vi "ALTS-2015-Read Serial Number.vi"(8 "error in (no error)":errorcluster) -> (0 "error out":errorcluster, 2 "Valid Serial Number?":bool, 3 "Serial No":string)   [LabVIEW 2013]
uses:
  Controls/ALTS-2015 LV2GBL Options.ctl
  Controls/ALTS-2015 Scanner Driver Options.ctl
  Misc/Controls/File Driver States.ctl
  OPC Engine/Controls/ALTS-2015 OPC Read Registers.ctl
  OPC Engine/Controls/ALTS-2015 OPC Read Global Options.ctl
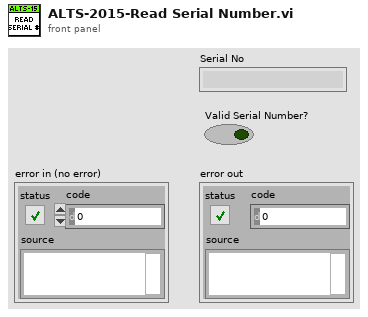
[diagram p1: front panel]
types:
  T1 = typedef "ALTS-2015 LV2GBL Options.ctl" = enum16{"Read all", "Write all"}
  T2 = typedef "ALTS-2015 INI Configuration Cluster.ctl" = cluster{"Application":cluster{"Rerun Count":i32, "Workorder No":string, "PLC Scanner":bool}, "Station Details":cluster{"Sensor Name 1":string, "Sensor Name 2":string, "Sensor Name 3":string, "Sensor Name 4":string, "Station1 Enable":bool, "Station2 Enable":bool, "Station3 Enable":bool, "Station4 Enable":bool}, "Database":cluster{"Database Connection Link":path, "Result Procedure":string, "User":string, "Password":string, "Prompt":bool, "Station 1 LT Result DB DSN Path":path, "Station 2 LT Result DB DSN Path":path, "Station 3 LT Result DB DSN Path":path, "Station 4 LT Result DB DSN Path":path, "AirLeakTestResult Procedure":string, "Serial Details Procedure":string}, "Simulation":cluster{"Simulate DAQ Hardware":bool, "Simulate Result DB Write":bool, "Simulate Scanner":bool, "Simulate OPC":bool, "Simulate Serial Details DB":bool, "Simulate Result DB":bool, "Simulate Scanner DB Path":path, "Simulate Serial Details DB Path":path, "Simulate Result DB Path":path}, "Barcode Scanner1":cluster{"Scanner IP":string, "Scanner Port":u16, "#Bytes to Read":i32, "Timeout_ms":i32}, "Barcode Scanner2":cluster{"Enabled?":bool, "Scanner IP":string, "Scanner Port":u16, "#Bytes to Read":i32}}
  T3 = typedef "File Driver States.ctl" = enum16{"Create/Open File", "Write File", "Close File"}
  T4 = typedef "ALTS-2015 Scanner Driver Options.ctl" = enum16{"Initialize Scanner", "Read Scanner", "Close Scanner"}
  T5 = typedef "ALTS-2015 OPC Read Global Options.ctl" = enum16{"Init", "Write Value", "Write Array", "Read Value", "Read Array", "Read All"}
  T6 = typedef "ALTS-2015 OPC Read Registers.ctl" = enum16{"Robot_Available", "Start_Test", "Stop_Test", "Scan_Trigger", "Station_No_Start_Stop_Test", "Scan_Serial_Number", "Robot_Restart", "Task_Pass", "Task_Failure"}
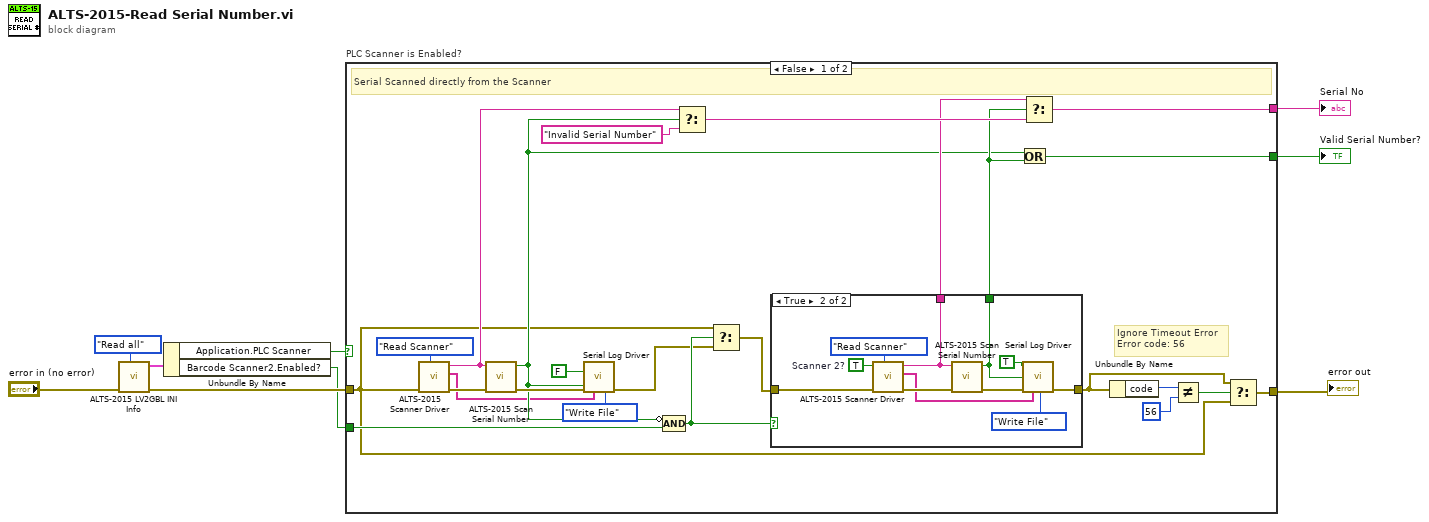
[diagram p0: block diagram]
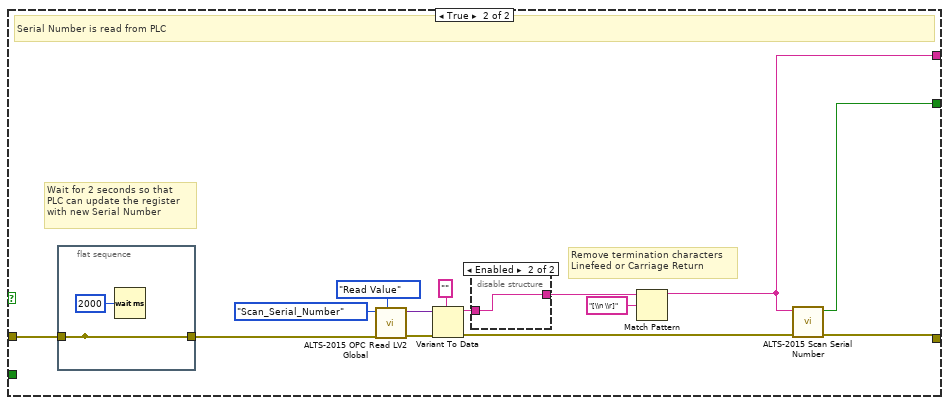
[diagram p3: hidden frame]
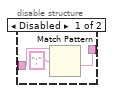
[diagram p4: hidden frame]
diagram:
  n1 = call "ALTS-2015 LV2GBL INI Info.vi"("Options"=ALTS-2015_LV2GBL_Options."Read all", "error in"="error in (no error)") -> ("error out"=w4:errorcluster, "Configuration Cluster Out"=w3:T2)  [unwired: 8 in]
  n2 = Unbundle By Name(w3) -> ("Application.PLC Scanner"=w2:bool, "Barcode Scanner2.Enabled?"=w1:bool)
  n3 = case "PLC Scanner is Enabled?" shown="False" w2 {
    tunnel: [w28 w48] -> w7
    tunnel: [w26 w49] -> w8
    tunnel: [w10 w47] -> w9
    tunnel: w4 -> [w11 w55]
    tunnel: w1 -> [w16 _]
    frame False {
      # "Ignore Timeout Error\nError code: 56"
      # "Serial Scanned directly from the Scanner"
      n4 = call "ALTS-2015 Scanner Driver.vi"("Operation"=ALTS-2015_Scanner_Driver_Options."Read Scanner", "error in (no error)"=w11) -> ("error out"=w33:errorcluster, "Serial Log Details"=w17:string[], "Serial No"=w29:string)  [unwired: 7 in]
      n5 = call "ALTS-2015 Scan Serial Number.vi"("error in"=w33, "Serial Number"=w29) -> ("error out"=w22:errorcluster, "Valid?"=w19:bool)  [unwired: 8 in]
      n6 = call "Serial Log Driver.vi"("Scanner 2?  (Scanner1)"=FALSE, "Valid Serial #"=w19, "error in (no error)"=w22, "Write Text"=w17, "operation"=File_Driver_States."Write File") -> ("error out"=w21:errorcluster)  [unwired: 10 in]
      n7 = Compound Arithmetic op=AND(invert w19, w16) -> (w24:bool)
      n8 = Select(t=w29, s=w19, f="Invalid Serial Number" ("Serial No")) -> (s? t:f=w32:string)
      n9 = Select(t=w11, s=w24, f=w21) -> (s? t:f=w23:errorcluster)
      n10 = case shown="True" w24 {
        tunnel: w23 -> [w34 w44]
        tunnel: [w34 w37] -> w12
        tunnel: [_ w36] -> w27
        tunnel: [_ w41] -> w30
        frame False {
        }
        frame True {
          w43 = TRUE  # Scanner 2?
          n11 = call "ALTS-2015 Scanner Driver.vi"("Operation"=ALTS-2015_Scanner_Driver_Options."Read Scanner", "error in (no error)"=w44, "Scanner 2?  (Scanner1)"=w43) -> ("error out"=w42:errorcluster, "Serial Log Details"=w35:string[], "Serial No"=w41:string)  [unwired: 6 in]
          n12 = call "ALTS-2015 Scan Serial Number.vi"("error in"=w42, "Serial Number"=w41) -> ("error out"=w39:errorcluster, "Valid?"=w36:bool)  [unwired: 8 in]
          n13 = call "Serial Log Driver.vi"("Scanner 2?  (Scanner1)"=TRUE, "Valid Serial #"=w36, "error in (no error)"=w39, "Write Text"=w35, "operation"=File_Driver_States."Write File") -> ("error out"=w37:errorcluster)  [unwired: 10 in]
        }
      }
      n14 = Or(x=w19, y=w27) -> (x .or. y?=w26:bool)
      n15 = Select(t=w30, s=w27, f=w32) -> (s? t:f=w28:string)
      n16 = Unbundle By Name(w12) -> ("code"=w13:i32)
      n17 = Not Equal?(x=w13, y=56) -> (x != y?=w15:bool)
      n18 = Select(t=w12, s=w15, f=w11) -> (s? t:f=w10:errorcluster)
    }
    frame True {
      # "Remove termination characters\nLinefeed or Carriage Return"
      # "Wait for 2 seconds so that \nPLC can update the register \nwith new Serial Number"
      # "Serial Number is read from PLC"
      n19 = flat-sequence {
        tunnel: w55 -> [w64]
        tunnel: [w64] -> _
        tunnel: [w64] -> w54
        frame #0 {
          n20 = Wait (ms)(milliseconds to wait=u32 2000) -> ()  [unwired: 1 out]
        }
      }
      n21 = call "ALTS-2015 OPC Read LV2 Global.vi"("Options"=ALTS-2015_OPC_Read_Global_Options."Read Value", "error in (no error)"=w54, "OPC Read Register"=ALTS-2015_OPC_Read_Registers."Scan_Serial_Number") -> ("error out"=w58:errorcluster, "OPC Read Reigter Value"=w59:variant)  [unwired: 6 in, 1 out]
      n22 = Variant To Data(error in=w58, type="", Variant=w59) -> (data=w51:string, error out=w50:errorcluster)
      n23 = disable-structure shown="Enabled" {
        disable-tunnel: [w61 w63] -> w52
        disable-tunnel: w51 -> [w60 w63]
        frame Disabled {
          n24 = Match Pattern(string=w60, regular expression=";") -> (after substring=w61:string)  [unwired: 1 in, 3 out]
        }
        frame Enabled {
        }
      }
      n25 = Match Pattern(string=w52, regular expression="[\\n \\r]") -> (before substring=w48:string)  [unwired: 1 in, 3 out]
      n26 = call "ALTS-2015 Scan Serial Number.vi"("error in"=w50, "Serial Number"=w48) -> ("error out"=w47:errorcluster, "Valid?"=w49:bool)  [unwired: 8 in]
    }
  }
  "error out" <- w9
  "Valid Serial Number?" <- w8
  "Serial No" <- w7
